vi "Suita SPAW7000 Range Test.vi"() -> ()   [LabVIEW 2018]
doc: "This example shows how to configure a range and check that the acquired measurements are within that range using the VIs of the driver."
uses:
  <instrlib>/Suita SPAW7000/Suita SPAW7000.lvlib
panel:
  out "Out of Range":bool
  in  "Lower Limit (-90.0 dBm)":dbl=-90.0 format="%#.6g"
  in  "Upper Limit (90.0 dBm)":dbl=90.0 format="%#.6g"
  in  "Timeout (10000 ms)":u32=10000
  out "Measurement":dbl
  in  "VISA resource name":refnum<visa-resource-name>
  # "(c) 2014 <Enter Company Name Here>.  ALL RIGHTS RESERVED."
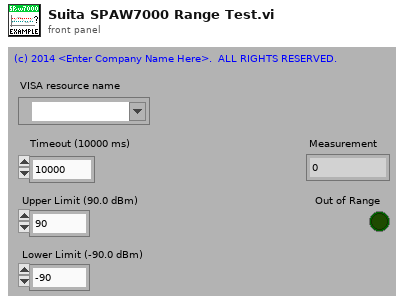
[diagram p1: front panel]
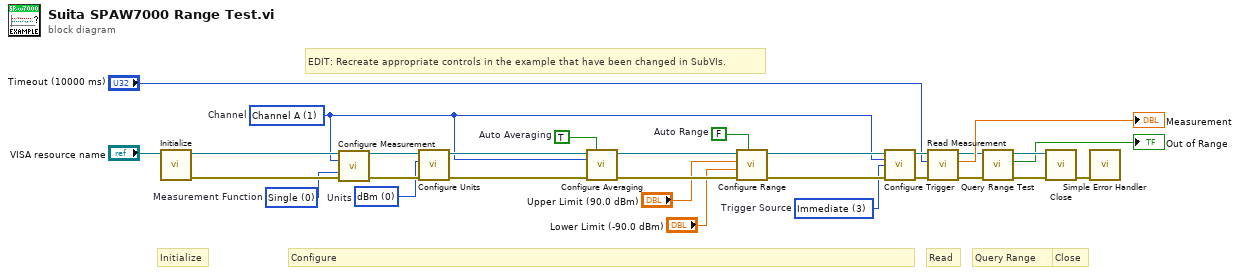
[diagram p0: block diagram]
diagram:
  w1 = u16 3 items=["Bus", "External", "Hold", "Immediate", "Internal A", "Internal B"]  # Trigger Source
  w10 = u16 0 items=["Single", "Difference", "Ratio"]  # Measurement Function
  w11 = u16 0 items=["dBm", "W"]  # Units
  w12 = TRUE  # Auto Averaging
  w13 = FALSE  # Auto Range
  w9 = u16 1 items=["Channel A"=1, "Channel B"=2]  # Channel
  # "EDIT: Recreate appropriate controls in the example that have been changed in SubVIs."
  # "Query Range"
  # "Close"
  # "Read"
  # "Configure"
  # "Initialize"
  n1 = call <instrlib>:"Initialize.vi"("VISA resource name"="VISA resource name") -> ("error out"=w29:errorcluster, "VISA resource name out"=w28:refnum<visa-resource-name>)  [unwired: 9 in]
  n2 = call <instrlib>:"Configure Measurement.vi"("VISA resource name"=w28, "First Channel (1: Channel A)"=w9, "Measurement Function (0: Single)"=w10, "error in (no error)"=w29) -> ("VISA resource name out"=w27:refnum<visa-resource-name>, "error out"=w26:errorcluster)  [unwired: 10 in]
  n3 = call <instrlib>:"Configure Units.vi"("error in (no error)"=w26, "Units (0: dBm)"=w11, "VISA resource name"=w27) -> ("error out"=w25:errorcluster, "VISA resource name out"=w24:refnum<visa-resource-name>)  [unwired: 7 in]
  n4 = call <instrlib>:"Configure Averaging.vi"("VISA resource name"=w24, "Auto Averaging (T: Enable)"=w12, "Channel (1: Channel A)"=w9, "error in (no error)"=w25) -> ("VISA resource name out"=w22:refnum<visa-resource-name>, "error out"=w23:errorcluster)  [unwired: 10 in]
  n5 = call <instrlib>:"Configure Range.vi"("Auto Range (T: Enable)"=w13, "error in (no error)"=w23, "Lower Limit (-90.0 dBm)"="Lower Limit (-90.0 dBm)", "Upper Limit (90.0 dBm)"="Upper Limit (90.0 dBm)", "VISA resource name"=w22) -> ("error out"=w21:errorcluster, "VISA resource name out"=w20:refnum<visa-resource-name>)  [unwired: 5 in]
  n6 = call <instrlib>:"Configure Trigger.vi"("VISA resource name"=w20, "Channel (1: Channel A)"=w9, "Trigger Source (3: Immediate)"=w1, "error in (no error)"=w21) -> ("VISA resource name out"=w19:refnum<visa-resource-name>, "error out"=w18:errorcluster)  [unwired: 10 in]
  n7 = call <instrlib>:"Read Measurement.vi"("error in (no error)"=w18, "Timeout (10000 ms)"="Timeout (10000 ms)", "VISA resource name"=w19) -> ("error out"=w3:errorcluster, "Measurement"=→"Measurement":dbl, "VISA resource name out"=w4:refnum<visa-resource-name>)  [unwired: 6 in]
  n8 = call <instrlib>:"Query Range Test.vi"("error in (no error)"=w3, "VISA resource name"=w4) -> ("error out"=w6:errorcluster, "Out of Range"=→"Out of Range":bool, "VISA resource name out"=w5:refnum<visa-resource-name>)  [unwired: 7 in]
  n9 = call <instrlib>:"Close.vi"("error in (no error)"=w6, "VISA resource name"=w5) -> ("error out"=w16:errorcluster)  [unwired: 9 in]
  n10 = call <vilib>:"Simple Error Handler.vi"("error in (no error)"=w16) -> ()  [unwired: 4 in, 5 out]
